vi "LSMcontroller_v56_from here for labview64bit.vi"() -> ()   [LabVIEW 2015] (continued)
                    n4807 = local read "wavdet"() -> (w1776:bool)
                    n4808 = call "correctwaveformsizetemp.vi"("new sampling frequency (Hz)"=w1773, "start"=FALSE, "reference waveforms to"=w1781, "Analog waveforms in"=w1788, "stop"=FALSE, "Digital waveforms in"=w1780) -> ("analog wf out"=w1784:waveform(dbl)[], "Digital wf out"=w1782:digitalwaveform[], "measpoints"=w1775:i32)
                    n4809 = local write "Analog Lines Plot"(w1784) -> ()
                    n4810 = call "GetNumCamFramesv2.vi"("Digital Waveform Graph"=w1782) -> ("Numeric"=w1783:i32)  [unwired: 10 in]
                    n4811 = local write "Digital Lines Plot"(w1782) -> ()
                    n4812 = case shown="True" w1776 {
                      tunnel: w1775 -> [_ w1796]
                      frame False {
                      }
                      frame True {
                        n4813 = local write "# of frames"(w1796) -> ()
                      }
                    }
                    n4814 = call "waveformsAObuffer.vi"("AO wf in"=w1784, "command"="set") -> ()  [unwired: 1 out]
                    n4815 = call "waveformsDObuffer.vi"("DO wf in"=w1782, "command"="set") -> ()  [unwired: 1 out]
                    n4816 = local write "Total Camera Frames"(w1783) -> ()
                  }
                }
              }
              frame #4 {
                n4817 = local read "finite samples"() -> (w1797:bool)
                n4818 = local read "continuous"() -> (w1798:bool)
                n4819 = local read "wavdet"() -> (w1799:bool)
                n4820 = call "2pparameters.vi"("command"="get") -> ("params out"=w1802:T12)  [unwired: 1 in]
                n4821 = Bundle By Name(cluster=w1802, "finite"=w1797, "cont"=w1798, "wavdet"=w1799) -> (w1800:T12)
                n4822 = call "2pparameters.vi"("Params in"=w1800, "command"="set") -> ()  [unwired: 1 out]
              }
            }
          }
          event "Add settings": Value Change {
            n4823 = event-data() -> ()  [unwired: 1 in, 6 out]
            n4824 = call "wfsettings.vi"("command"="get") -> ("wfsettings out"=w1806:T29)  [unwired: 2 in, 1 out]
            n4825 = in-place {
              n4826 = in-place-cluster #53(w1806) -> ("settings names"=w1811:string[], "settings locations"=w1813:path[])
              n4827 = local read "Setting location"() -> (w1809:path)
              n4828 = local read "Nickname"() -> (w1808:string)
              n4829 = Build Array (concatenate)(w1811, w1808) -> (w1810:string[])
              n4830 = property on="Loaded settings" class="Ring (strict)"("Strings []"=w1810) -> ()  [unwired: 2 in, 2 out]
              n4831 = Build Array (concatenate)(w1813, w1809) -> (w1812:path[])
              n4832 = in-place-cluster #53("settings names"=w1810, "settings locations"=w1812) -> (w1804:T29)
            }
            n4833 = call "wfsettings.vi"("wfsettings in"=w1804, "command"="set") -> ()  [unwired: 1 in, 2 out]
          }
          event "Rem setting": Value Change {
            n4834 = event-data() -> ()  [unwired: 1 in, 6 out]
            n4835 = call "wfsettings.vi"("command"="get") -> ("wfsettings out"=w1816:T29)  [unwired: 2 in, 1 out]
            n4836 = in-place {
              n4837 = in-place-cluster #54(w1816) -> ("settings names"=w1821:string[], "settings locations"=w1819:path[])
              n4838 = property on="Loaded settings" class="Ring (strict)"() -> ("RingText.Text"=w1822:string)  [unwired: 2 in, 2 out]
              n4839 = Search 1D Array(1D array=w1821, element=w1822) -> (index of element=w1823:i32)  [unwired: 1 in]
              n4840 = Delete From Array(array=w1821, index=w1823) -> (array with subset deleted=w1820:string[])  [unwired: 1 in, 1 out]
              n4841 = Delete From Array(array=w1819, index=w1823) -> (array with subset deleted=w1818:path[])  [unwired: 1 in, 1 out]
              n4842 = property on="Loaded settings" class="Ring (strict)"("Strings []"=w1820) -> ()  [unwired: 2 in, 2 out]
              n4843 = in-place-cluster #54("settings names"=w1820, "settings locations"=w1818) -> (w1814:T29)
            }
            n4844 = call "wfsettings.vi"("wfsettings in"=w1814, "command"="set") -> ()  [unwired: 1 in, 2 out]
          }
          event "Update settings": Value Change {
            n4845 = event-data() -> ()  [unwired: 1 in, 6 out]
            n4846 = stacked-sequence {
              frame #0 {
                n4847 = local read "Measurement"() -> (w1824:T5)
                n4848 = case shown="\"Timetrace\"" w1824 {
                  frame "X-Y-t movie", Default {
                    n4849 = local read "avpp"() -> (w1845:i32)
                    n4850 = local read "Angle ref"() -> (w1844:dbl)
                    n4851 = local read "ROI Type"() -> (w1843:u16)
                    n4852 = local read "xpixels ref"() -> (w1840:i32)
                    n4853 = local read "Vx-min ref"() -> (w1839:dbl)
                    n4854 = local read "Vx-max ref"() -> (w1838:dbl)
                    n4855 = local read "ypixels ref"() -> (w1836:i32)
                    n4856 = local read "Vy-min ref"() -> (w1837:dbl)
                    n4857 = local read "Vy-max ref"() -> (w1833:dbl)
                    n4858 = local read "Sampling rate"() -> (w1827:dbl)
                    n4859 = local read "finite samples"() -> (w1828:bool)
                    n4860 = local read "continuous"() -> (w1831:bool)
                    n4861 = local read "wavdet"() -> (w1832:bool)
                    n4862 = local read "# of frames"() -> (w1830:i32)
                    n4863 = local read "maxbufferAI"() -> (w1829:i32)
                    n4864 = local read "Override AI buffer"() -> (w1825:bool)
                    n4865 = call "2pparameters.vi"("command"="get") -> ("params out"=w1842:T12)  [unwired: 1 in]
                    n4866 = Bundle By Name(cluster=w1842, "type"="X-Y-t movie", "avpp"=w1845, "Angle Img"=w1844, "Xpixels Img"=w1840, "Vx-min Img"=w1839, "VX-max Img"=w1838, "Ypixels Img"=w1836, "Vy-min Img"=w1837, "Vy-max Img"=w1833, "srate"=w1827, "srate Img"=w1827, "finite"=w1828, "cont"=w1831, "wavdet"=w1832, "measpoints"=w1830, "maxbufferAI"=w1829, "Drawing Mode"=w1843, "Vz-reset"=0.0, "AIoverride"=w1825) -> (w1834:T12)
                    n4867 = call "2pparameters.vi"("Params in"=w1834, "command"="set") -> ()  [unwired: 1 out]
                  }
                  frame "X-Y-Z stack" {
                    n4868 = call "2pparameters.vi"("command"="get") -> ("params out"=w1849:T12)  [unwired: 1 in]
                    n4869 = Bundle By Name(cluster=w1849, "type"="X-Y-Z stack") -> (w1847:T12)
                    n4870 = call "2pparameters.vi"("Params in"=w1847, "command"="set") -> ()  [unwired: 1 out]
                  }
                  frame "Lifetime (scan)" {
                    n4871 = call "2pparameters.vi"("command"="get") -> ("params out"=w1854:T12)  [unwired: 1 in]
                    n4872 = Bundle By Name(cluster=w1854, "type"="Lifetime (scan)") -> (w1852:T12)
                    n4873 = call "2pparameters.vi"("Params in"=w1852, "command"="set") -> ()  [unwired: 1 out]
                  }
                  frame "Lifetime (contour)" {
                    n4874 = local read "Vy-min draw"() -> (w1864:dbl)
                    n4875 = local read "Vy-max draw"() -> (w1863:dbl)
                    n4876 = local read "Vx-min draw"() -> (w1866:dbl)
                    n4877 = local read "Vx-max draw"() -> (w1865:dbl)
                    n4878 = local read "xpixels ref"() -> (w1862:i32)
                    n4879 = local read "ypixels ref"() -> (w1861:i32)
                    n4880 = local read "ROI Type"() -> (w1860:u16)
                    n4881 = local read "srateAODOtt"() -> (w1871:dbl)
                    n4882 = local read "# of frames"() -> (w1876:i32)
                    n4883 = local read "refreshtime"() -> (w1868:dbl)
                    n4884 = local read "Pel"() -> (w1859:dbl)
                    n4885 = local read "bin"() -> (w1874:dbl)
                    n4886 = local read "Override AI buffer"() -> (w1857:bool)
                    n4887 = local read "finite samples"() -> (w1883:bool)
                    n4888 = local read "srateAODOtt"() -> (w1870:dbl)
                    n4889 = local read "srateAODOtt"() -> (w1877:dbl)
                    n4890 = local read "continuous"() -> (w1882:bool)
                    n4891 = local read "Angle ref"() -> (w1867:dbl)
                    n4892 = local read "wavdet"() -> (w1884:bool)
                    n4893 = local read "Vx-ref"() -> (w1879:dbl)
                    n4894 = local read "Vy-ref"() -> (w1881:dbl)
                    n4895 = local read "avpp"() -> (w1880:i32)
                    n4896 = call "tt_timeandsamples.vi"("bin"=w1874, "refreshtime"=w1868, "srateAODOtt"=w1871, "tot#ofsamples"=w1876) -> ("refreshrate"=w1872:dbl, "refreshbuffer"=w1873:i32, "timetracecycles"=w1878:i32)  [unwired: 5 in]
                    n4897 = local read "bin"() -> (w1875:dbl)
                    n4898 = call "2pparameters.vi"("command"="get") -> ("params out"=w1887:T12)  [unwired: 1 in]
                    n4899 = Bundle By Name(cluster=w1887, "Drawing Mode"=w1860, "measpoints"=w1876, "tt_cycles"=w1878, "refreshbuffer"=w1873, "refreshrate"=w1872, "Vx-ref"=w1879, "Vy-ref"=w1881, "srate"=w1870, "finite"=w1883, "cont"=w1882, "wavdet"=w1884, "avpp"=w1880, "srateAODO"=w1877, "bufferAI"=w1873, "bin"=w1875, "Angle Img"=w1867, "Vxminref"=w1866, "Vxmaxref"=w1865, "Vyminref"=w1864, "Vymaxref"=w1863, "Xpixels Img"=w1862, "Ypixels Img"=w1861, "Pel"=w1859, "Vz-reset"=0.0, "AIoverride"=w1857, "type"="Lifetime (contour)") -> (w1885:T12)
                    n4900 = Reciprocal(x=w1872) -> (1/x=w1869:dbl)
                    n4901 = local write "refreshtime"(w1869) -> ()
                    n4902 = call "2pparameters.vi"("Params in"=w1885, "command"="set") -> ()  [unwired: 1 out]
                  }
                  frame "X-Y-Z-t movie" {
                  }
                  frame "linescan" {
                  }
                  frame "Timetrace" {
                    n4903 = local read "Vy-min draw"() -> (w1897:dbl)
                    n4904 = local read "Vy-max draw"() -> (w1896:dbl)
                    n4905 = local read "Vx-min draw"() -> (w1899:dbl)
                    n4906 = local read "Vx-max draw"() -> (w1898:dbl)
                    n4907 = local read "xpixels ref"() -> (w1895:i32)
                    n4908 = local read "ypixels ref"() -> (w1894:i32)
                    n4909 = local read "ROI Type"() -> (w1893:u16)
                    n4910 = local read "srateAODOtt"() -> (w1904:dbl)
                    n4911 = local read "# of frames"() -> (w1909:i32)
                    n4912 = local read "refreshtime"() -> (w1901:dbl)
                    n4913 = local read "Pel"() -> (w1892:dbl)
                    n4914 = local read "bin"() -> (w1907:dbl)
                    n4915 = local read "Override AI buffer"() -> (w1890:bool)
                    n4916 = local read "finite samples"() -> (w1916:bool)
                    n4917 = local read "srateAODOtt"() -> (w1903:dbl)
                    n4918 = local read "srateAODOtt"() -> (w1910:dbl)
                    n4919 = local read "continuous"() -> (w1915:bool)
                    n4920 = local read "Angle ref"() -> (w1900:dbl)
                    n4921 = local read "wavdet"() -> (w1917:bool)
                    n4922 = local read "Vx-ref"() -> (w1912:dbl)
                    n4923 = local read "Vy-ref"() -> (w1914:dbl)
                    n4924 = local read "avpp"() -> (w1913:i32)
                    n4925 = call "tt_timeandsamples.vi"("bin"=w1907, "refreshtime"=w1901, "srateAODOtt"=w1904, "tot#ofsamples"=w1909) -> ("refreshrate"=w1905:dbl, "refreshbuffer"=w1906:i32, "timetracecycles"=w1911:i32)  [unwired: 5 in]
                    n4926 = local read "bin"() -> (w1908:dbl)
                    n4927 = call "2pparameters.vi"("command"="get") -> ("params out"=w1920:T12)  [unwired: 1 in]
                    n4928 = Bundle By Name(cluster=w1920, "Drawing Mode"=w1893, "measpoints"=w1909, "tt_cycles"=w1911, "refreshbuffer"=w1906, "refreshrate"=w1905, "Vx-ref"=w1912, "Vy-ref"=w1914, "srate"=w1903, "finite"=w1916, "cont"=w1915, "wavdet"=w1917, "avpp"=w1913, "srateAODO"=w1910, "bufferAI"=w1906, "bin"=w1908, "Angle Img"=w1900, "Vxminref"=w1899, "Vxmaxref"=w1898, "Vyminref"=w1897, "Vymaxref"=w1896, "Xpixels Img"=w1895, "Ypixels Img"=w1894, "Pel"=w1892, "Vz-reset"=0.0, "AIoverride"=w1890, "type"="Timetrace") -> (w1918:T12)
                    n4929 = Reciprocal(x=w1905) -> (1/x=w1902:dbl)
                    n4930 = local write "refreshtime"(w1902) -> ()
                    n4931 = call "2pparameters.vi"("Params in"=w1918, "command"="set") -> ()  [unwired: 1 out]
                  }
                  frame "Lifetime (point)" {
                  }
                }
              }
              frame #1 {
                w1923 = FALSE ("wavdet")
                n4932 = call "2pparameters.vi"("command"="get") -> ("params out"=w1927:T12)  [unwired: 1 in]
                n4933 = Bundle By Name(cluster=w1927, "finite"=w1923, "cont"=w1923, "wavdet"=TRUE) -> (w1924:T12)
                n4934 = call "2pparameters.vi"("Params in"=w1924, "command"="set") -> ()  [unwired: 1 out]
              }
              frame #2 {
                n4935 = property on="Loaded settings" class="Ring (strict)"() -> ("RingText.Text"=w1929:string)  [unwired: 2 in, 2 out]
                n4936 = control-ref of="Analog Lines Plot"() -> (w1931:refnum<vi>)
                n4937 = control-ref of="Digital Lines Plot"() -> (w1930:refnum<vi>)
                n4938 = call "Usedlinesfromsettingsfile.vi"("sertting"=w1929) -> ("used AO names"=w1935:string[], "used AO lines"=w1934:tag[], "used DO names"=w1933:string[], "used DO lines"=w1932:tag[])
                n4939 = call "loadAODOwfparamsfromsettingsfile.vi"("sertting"=w1929) -> ()
                n4940 = call "prepAOWaveplot.vi"("WaveformGraph in"=w1931, "Analog Used Names"=w1935) -> ()  [unwired: 1 in]
                n4941 = local write "Analog Used Names"(w1935) -> ()
                n4942 = local write "Analog Used Lines"(w1934) -> ()
                n4943 = call "prepDOWaveplot.vi"("DigitalGraph in"=w1930, "used DO names"=w1933) -> ()  [unwired: 1 in]
                n4944 = local write "Digital Used Names"(w1933) -> ()
                n4945 = local write "Digital Used Lines"(w1932) -> ()
              }
              frame #3 {
                n4946 = call "waveformparamsv2.vi"("command"="get") -> ("Params out"=w1952:T16)  [unwired: 4 in, 2 out]
                n4947 = Unbundle By Name(w1952) -> ("AO parameters"=w1953:T17, "DO parameters"=w1954:T19)
                n4948 = for {
                  tunnel: w1953 -> [w1973] mode=indexing
                  tunnel: [w1971] -> w1955 mode=indexing
                  tunnel: [w1970] -> w1940 mode=indexing
                  tunnel: [w1968] -> w1943 mode=indexing
                  i -> [w1972]
                  n4949 = Unbundle By Name(w1973) -> ("AOtab"=w1974:dbl)
                  n4950 = case shown="0, Default" w1974 {
                    tunnel: w1973 -> [_ w1985 w1987 w1989]
                    tunnel: [_ w1984 w1986 w1988] -> w1969
                    frame -1 {
                    }
                    frame 0, Default {
                      n4951 = call "generateRampedSquareWave_fromAOparameters.vi"("AO params"=w1985) -> ("Waveform"=w1984:waveform(dbl))  [unwired: 1 out]
                    }
                    frame 1 {
                      n4952 = call "generateTriWave_fromAOparameters.vi"("AO params"=w1987) -> ("Waveform"=w1986:waveform(dbl))  [unwired: 1 out]
                    }
                    frame 2 {
                      n4953 = call "matlabAOwffromparam.vi"("Cluster"=w1989) -> ("Waveform"=w1988:waveform(dbl))  [unwired: 1 out]
                    }
                  }
                  n4954 = case shown="0" w1972 {
                    tunnel: [w1979 -1] -> w1971
                    tunnel: [w1978 w1982] -> w1970
                    tunnel: w1969 -> [w1978 w1982]
                    tunnel: [w1975 -1.0] -> w1968
                    frame 0 {
                      n4955 = Unbundle By Name(w1978) -> ("dt"=w1977:dbl, "Y"=w1980:dbl[])
                      n4956 = Reciprocal(x=w1977) -> (1/x=w1976:dbl)
                      n4957 = Array Size(array=w1980) -> (size(s)=w1979:i32)
                      n4958 = Round To Nearest(number=w1976) -> (nearest integer value=w1975:dbl)
                    }
                    frame 1, Default {
                    }
                  }
                }
                n4959 = Index Array(array=w1955, index=0) -> (element=w1957:i32)
                n4960 = Index Array(array=w1943, index=0) -> (element=w1942:dbl)
                n4961 = for {
                  tunnel: w1954 -> [w1962] mode=indexing
                  tunnel: [w1960] -> w1941 mode=indexing
                  tunnel: w1957 -> [w1959]
                  n4962 = Unbundle By Name(w1962) -> ("DOtab"=w1961:dbl)
                  n4963 = case shown="0, Default" w1961 {
                    tunnel: w1962 -> [w1965 w1967]
                    tunnel: w1959 -> [w1964 _]
                    tunnel: [w1963 w1966] -> w1960
                    frame 0, Default {
                      n4964 = call "simple digital from wf params.vi"("waveform params"=w1965, "number of samples"=w1964) -> ("digital waveform"=w1963:digitalwaveform)
                    }
                    frame 1 {
                      n4965 = call "matlabDOwffromparam.vi"("waveform params"=w1967) -> ("digital waveform"=w1966:digitalwaveform)
                    }
                  }
                }
                n4966 = property on="refwf" class="Ring (strict)"() -> ("RingText.Text"=w1945:string)  [unwired: 2 in, 2 out]
                n4967 = call "correctwaveformsizetemp.vi"("new sampling frequency (Hz)"=w1942, "start"=FALSE, "reference waveforms to"=w1945, "Analog waveforms in"=w1940, "stop"=FALSE, "Digital waveforms in"=w1941) -> ("analog wf out"=w1939:waveform(dbl)[], "Digital wf out"=w1938:digitalwaveform[], "measpoints"=w1936:i32)
                n4968 = local read "wavdet"() -> (w1937:bool)
                n4969 = case shown="True" w1937 {
                  tunnel: w1936 -> [_ w1958]
                  frame False {
                  }
                  frame True {
                    n4970 = local write "# of frames"(w1958) -> ()
                  }
                }
                n4971 = local write "Analog Lines Plot"(w1939) -> ()
                n4972 = local write "Digital Lines Plot"(w1938) -> ()
                n4973 = call "GetNumCamFramesv2.vi"("Digital Waveform Graph"=w1938) -> ("Numeric"=w1950:i32)  [unwired: 10 in]
                n4974 = call "waveformsAObuffer.vi"("AO wf in"=w1939, "command"="set") -> ()  [unwired: 1 out]
                n4975 = call "waveformsDObuffer.vi"("DO wf in"=w1938, "command"="set") -> ()  [unwired: 1 out]
                n4976 = local write "Total Camera Frames"(w1950) -> ()
              }
              frame #4 {
                n4977 = local read "AO channels"() -> (w1990:u32)
                n4978 = call "2pparameters.vi"("command"="get") -> ("params out"=w1992:T12)  [unwired: 1 in]
                n4979 = Unbundle By Name(w1992) -> ("aAO"=w1991:u32[])
                n4980 = Search 1D Array(1D array=w1991, element=w1990) -> (index of element=w1994:i32)  [unwired: 1 in]
                n4981 = Equal?(x=w1994, y=-1.0) -> (x = y?=w1995:bool)
                n4982 = case shown="False" w1995 {
                  tunnel: w1994 -> [w2020 _]
                  frame False {
                    n4983 = call "waveformparamsv2.vi"("command"="get") -> ("Params out"=w2003:T16)  [unwired: 4 in, 2 out]
                    n4984 = Unbundle By Name(w2003) -> ("AO parameters"=w2002:T17)
                    n4985 = Index Array(array=w2002, index=w2020) -> (element=w2019:T18)
                    n4986 = Unbundle By Name(w2019) -> ("AOtab"=w2000:dbl, "Repeats"=w2018:dbl, "Cycles"=w2017:dbl, "Start amplitude (V)"=w2016:dbl, "Baseline (V)"=w2015:dbl, "Step size (V)"=w2014:dbl, "DC (%)"=w2013:dbl, "Sampling frequency (Hz)"=w2012:dbl, "Period (ms)"=w2011:dbl, "Offset (V)"=w2010:dbl, "Amplitude (V)"=w2009:dbl, "Frequency"=w2008:dbl, "Tri Repeats"=w2007:dbl, "phase shift (ms)"=w2006:dbl, "Pulses"=w2005:dbl, "Tri phase"=w2001:dbl, "padding value"=w1997:dbl, "Matlab wave file"=w1998:path)
                    n4987 = To Unsigned Long Integer(number=w2000) -> (unsigned 32bit integer=w1999:u32)
                    n4988 = local write "Build analog waveform tabs"(w1999) -> ()
                    n4989 = local write "Matlab waveform path"(w1998) -> ()
                    n4990 = local write "phase shift (ms)"(w2006) -> ()
                    n4991 = local write "Repeats"(w2018) -> ()
                    n4992 = local write "Cycles"(w2017) -> ()
                    n4993 = local write "Amplitude (V)"(w2009) -> ()
                    n4994 = local write "Matlab padding value"(w1997) -> ()
                    n4995 = local write "Tri padding value"(w1997) -> ()
                    n4996 = local write "Start amplitude (V)"(w2016) -> ()
                    n4997 = local write "Tri Phase (s)"(w2001) -> ()
                    n4998 = local write "Period (ms)"(w2011) -> ()
                    n4999 = local write "Tri Repeats"(w2007) -> ()
                    n5000 = local write "Offset (V)"(w2010) -> ()
                    n5001 = local write "Frequency"(w2008) -> ()
                    n5002 = local write "Pulses"(w2005) -> ()
                    n5003 = local write "padding value"(w1997) -> ()
                    n5004 = local write "Sampling rate \ncurrent wf"(w2012) -> ()
                    n5005 = local write "Baseline (V)"(w2015) -> ()
                    n5006 = local write "Step size (V)"(w2014) -> ()
                    n5007 = local write "DC (%)"(w2013) -> ()
                  }
                  frame True {
                  }
                }
              }
              frame #5 {
                n5008 = local read "DO channels"() -> (w2023:u16)
                n5009 = call "2pparameters.vi"("command"="get") -> ("params out"=w2025:T12)  [unwired: 1 in]
                n5010 = Unbundle By Name(w2025) -> ("aDO"=w2024:u32[])
                n5011 = Search 1D Array(1D array=w2024, element=w2023) -> (index of element=w2022:i32)  [unwired: 1 in]
                n5012 = Equal?(x=w2022, y=-1.0) -> (x = y?=w2021:bool)
                n5013 = case shown="False" w2021 {
                  tunnel: w2022 -> [w2040 _]
                  frame False {
                    n5014 = call "waveformparamsv2.vi"("command"="get") -> ("Params out"=w2034:T16)  [unwired: 4 in, 2 out]
                    n5015 = Unbundle By Name(w2034) -> ("DO parameters"=w2032:T19)
                    n5016 = Index Array(array=w2032, index=w2040) -> (element=w2039:T20)
                    n5017 = Unbundle By Name(w2039) -> ("Digital DC (%)"=w2038:dbl, "Digital phase"=w2037:dbl, "Digital Freq (Hz)"=w2036:dbl, "Sampling frequency (Hz)"=w2035:dbl, "Digital time offset (s)"=w2031:dbl, "padding value"=w2030:dbl, "matlab wave file"=w2029:path, "DOtab"=w2028:dbl)
                    n5018 = local write "Build digital waveform tabs"(w2028) -> ()
                    n5019 = local write "Digital DC (%)"(w2038) -> ()
                    n5020 = local write "Matlab waveform path DO"(w2029) -> ()
                    n5021 = local write "Sampling rate \ncurrent wf"(w2035) -> ()
                    n5022 = local write "Digital time offset (s)"(w2031) -> ()
                    n5023 = local write "Matlab padding value DO"(w2030) -> ()
                    n5024 = local write "Digital padding value"(w2030) -> ()
                    n5025 = local write "Digital Freq (Hz)"(w2036) -> ()
                    n5026 = local write "Digital phase (s)"(w2037) -> ()
                  }
                  frame True {
                  }
                }
              }
              frame #6 {
                n5027 = local read "finite samples"() -> (w2041:bool)
                n5028 = local read "continuous"() -> (w2042:bool)
                n5029 = local read "wavdet"() -> (w2043:bool)
                n5030 = call "2pparameters.vi"("command"="get") -> ("params out"=w2046:T12)  [unwired: 1 in]
                n5031 = Bundle By Name(cluster=w2046, "finite"=w2041, "cont"=w2042, "wavdet"=w2043) -> (w2044:T12)
                n5032 = call "2pparameters.vi"("Params in"=w2044, "command"="set") -> ()  [unwired: 1 out]
              }
            }
          }
          event "Exit": Value Change {
            n5033 = event-data() -> ("NewVal"=w2048:bool)  [unwired: 1 in]
          }
        }
        n5034 = Wait (ms)(milliseconds to wait=u32 50) -> ()  [unwired: 1 out]
      }
    }
    frame #3 {
      w6436 = u16 1 items=["OD 0"=1, "OD 0.5"=2, "OD 1"=3, "OD 2"=4, "OD 3"=5, "OD 4"=6] ("New ODfilt")
      w6438 = FALSE ("Value (Signaling)")
      n5035 = property on="Start" class="Bool (strict)"("Val(Sgnl)"=w6438) -> ()  [unwired: 2 in, 2 out]
      n5036 = property on="Exit" class="Bool (strict)"("Val(Sgnl)"=w6438) -> ()  [unwired: 2 in, 2 out]
      n5037 = property on="Stop" class="Bool (strict)"("Val(Sgnl)"=w6438) -> ()  [unwired: 2 in, 2 out]
      n5038 = local read "ODfilt"() -> (w6437:u16)
      n5039 = call "filterwheelcontrol_nothorlabslib.vi"("Current OD filt"=w6437, "New ODfilt"=w6436) -> ()  [unwired: 1 in]
    }
  }
